vi "Receiver.vi"() -> ()   [LabVIEW 2015]
uses:
  <instrlib>/niUSRP/niUSRP Fetch Rx Data (CDB WDT).vi
panel:
  out "Demodulated Square":dbl(graph)
  in  "stop":bool
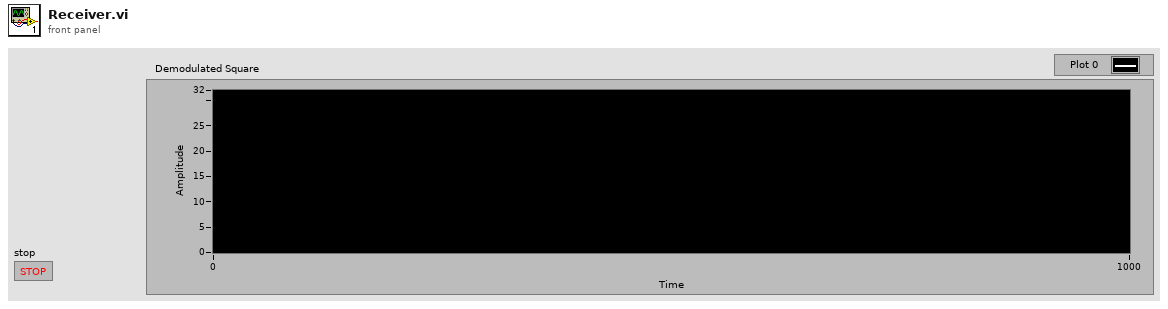
[diagram p1: front panel]
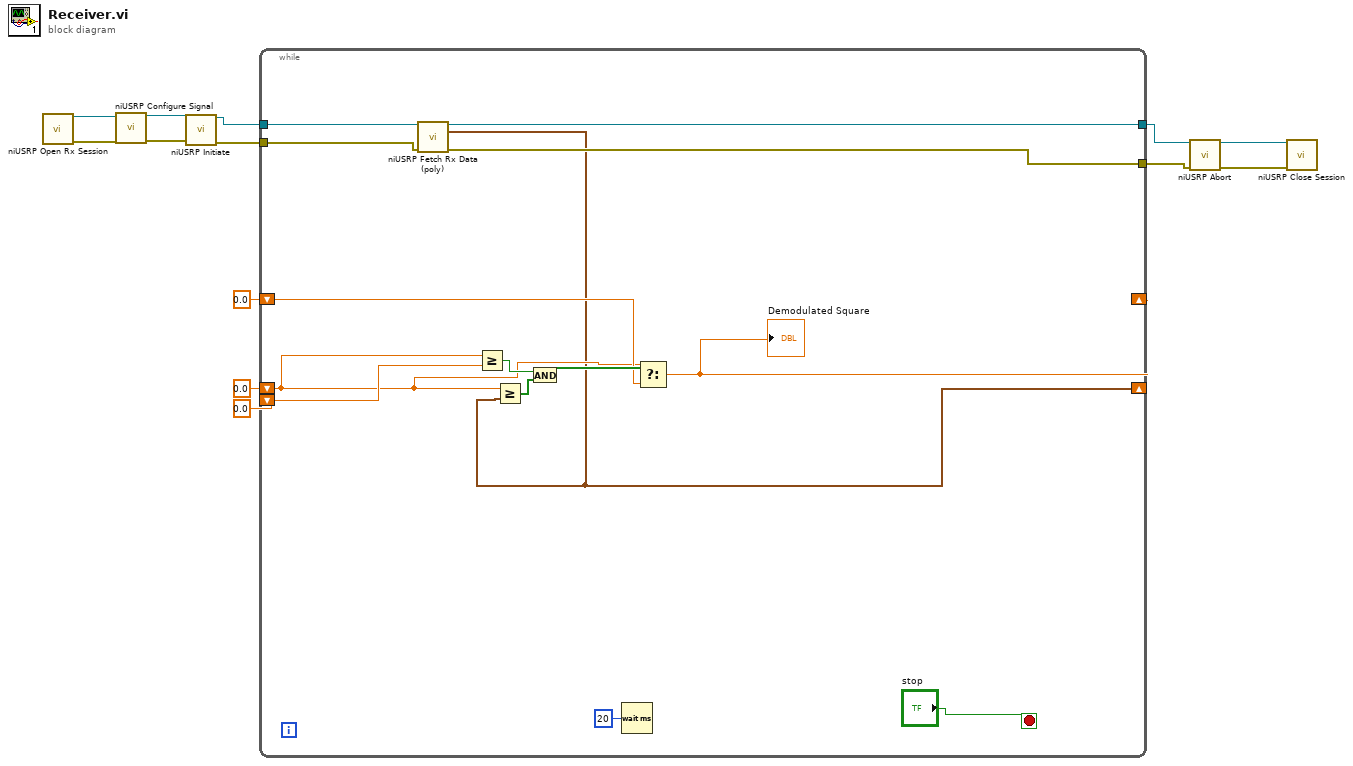
[diagram p0: block diagram]
diagram:
  n1 = call <instrlib>:"niUSRP Open Rx Session.vi"() -> ("session handle out"=w5:refnum<k15>, "error out"=w10:errorcluster)  [unwired: 14 in]
  n2 = call <instrlib>:"niUSRP Configure Signal.vi"("session handle"=w5, "error in (no error)"=w10) -> ("session handle out"=w4:refnum<k15>, "error out"=w9:errorcluster)  [unwired: 9 in, 3 out]
  n3 = call <instrlib>:"niUSRP Initiate.vi"("session handle"=w4, "error in (no error)"=w9) -> ("session handle out"=w3:refnum<k15>, "error out"=w8:errorcluster)  [unwired: 12 in]
  n4 = while {
    shift-right: [w14] -> _
    shift-left: 0.0 -> [w15]
    shift-left: 0.0 -> [w25]
    shift-right: [w21] -> _
    shift-left: 0.0 -> [w22]
    tunnel: w8 -> [w20]
    tunnel: [w19] -> w7
    tunnel: w3 -> [w18]
    tunnel: [w17] -> w2
    stop <- "stop" stop-if-true
    n5 = call-poly <instrlib>:"niUSRP Fetch Rx Data (poly).vi"("session handle"=w18, "error in (no error)"=w20) -> ("session handle out"=w17:refnum<k15>, "data"=w14:waveform(cdb), "error out"=w19:errorcluster)  [unwired: 10 in, 1 out]
    n6 = Greater Or Equal?(x=w15, y=w25) -> (x >= y?=w24:bool)
    n7 = Greater Or Equal?(x=w15, y=w14) -> (x >= y?=w16:bool[])
    n8 = And(x=w24, y=w16) -> (x .and. y?=w23:bool[])
    n9 = Wait (ms)(milliseconds to wait=u32 20) -> ()  [unwired: 1 out]
    n10 = Select(t=w15, s=w23, f=w22) -> (s? t:f=w21:dbl)
    "Demodulated Square" <- w21
  }
  n11 = call <instrlib>:"niUSRP Abort.vi"("session handle"=w2, "error in (no error)"=w7) -> ("session handle out"=w1:refnum<k15>, "error out"=w6:errorcluster)  [unwired: 12 in]
  n12 = call <instrlib>:"niUSRP Close Session.vi"("session handle"=w1, "error in (no error)"=w6) -> ()  [unwired: 13 in, 1 out]
